vi "test_read-nmea-data2.vi"() -> ()   [LabVIEW 2019] (continued)
11,72,359,29,7*79\n\t\n15:13:14.60\tF9P\t$GAGSV,2,2,08,12,40,103,25,19,26,045,19,25,09,249,,36,26,308,17,7*71\n\t\n15:13:14.62\tF9P\t$GAGSV,2,1,08,02,08,297,,04,66,116,25,09,32,193,,11,72,359,,2*77\n\t\n15:13:14.64\tF9P\t$GAGSV,2,2,08,12,40,103,,19,26,045,,25,09,249,,36,26,308,,2*7D\n\t\n15:13:14.66\tF9P\t$GBGSV,1,1,04,11,49,132,31,14,87,114,29,28,,,21,33,61,220,31,1*44\n\t\n15:13:14.68\tF9P\t$GBGSV,1,1,03,11,49,132,28,14,87,114,,33,61,220,,3*49\n\t\n15:13:14.70\tF9P\t$GNGLL,3723.55651,N,12656.97723,E,061316.00,A,A*7D\n\t\n15:13:14.72\tF9P\t\t\n15:13:14.74\tF9P\t\t\n15:13:14.76\tF9P\t\t\n15:13:14.78\tF9P\t\t\n15:13:14.80\tF9P\t\t\n15:13:14.82\tF9P\t\t\n15:13:14.84\tF9P\t\t\n15:13:14.86\tF9P\t\t\n15:13:14.88\tF9P\t\t\n15:13:14.90\tF9P\t\t\n15:13:14.92\tF9P\t\t\n15:13:14.94\tF9P\t\t\n15:13:14.96\tF9P\t\t\n15:13:14.98\tF9P\t\t\n15:13:15.00\tF9P\t\t\n15:13:15.02\tF9P\t\t\n15:13:15.04\tF9P\t\t\n15:13:15.06\tF9P\t\t\n15:13:15.08\tF9P\t\t\n15:13:15.10\tF9P\t\t\n15:13:15.12\tF9P\t\t\n15:13:15.14\tF9P\t\t\n15:13:15.16\tF9P\t\t\n15:13:15.18\tF9P\t\t\n15:13:15.20\tF9P\t\t\n15:13:15.22\tF9P\t\t\n15:13:15.24\tF9P\t$GNRMC,061317.00,A,3723.55689,N,12656.97802,E,2.086,57.57,250720,,,A,V*36\n\t\n15:13:15.26\tF9P\t$GNVTG,57.57,T,,M,2.086,N,3.863,K,A*11\n\t\n15:13:15.28\tF9P\t$GNGGA,061317.00,3723.55689,N,12656.97802,E,1,12,0.86,49.2,M,18.5,M,,*7E\n\t\n15:13:15.30\tF9P\t$GNGSA,A,3,12,06,19,05,17,09,04,02,,,,,1.43,0.86,1.13,1*0B\n\t\n15:13:15.32\tF9P\t$GNGSA,A,3,85,70,71,84,,,,,,,,,1.43,0.86,1.13,2*09\n\t\n15:13:15.34\tF9P\t$GNGSA,A,3,36,19,11,04,09,12,,,,,,,1.43,0.86,1.13,3*0B\n\t\n15:13:15.36\tF9P\t$GNGSA,A,3,14,11,33,,,,,,,,,,1.43,0.86,1.13,4*0A\n\t\n15:13:15.38\tF9P\t$GPGSV,3,1,09,02,55,319,24,04,18,043,23,05,37,247,29,06,64,049,30,1*6A\n\t\n15:13:15.40\tF9P\t$GPGSV,3,2,09,09,45,074,36,12,23,276,22,17,33,154,36,19,52,157,32,1*6D\n\t\n15:13:15.42\tF9P\t$GPGSV,3,3,09,25,12,306,19,1*54\n\t\n15:13:15.44\tF9P\t$GPGSV,3,1,09,02,55,319,,04,18,043,16,05,37,247,24,06,64,049,23,6*62\n\t\n15:13:15.46\tF9P\t$GPGSV,3,2,09,09,45,074,27,12,23,276,,17,33,154,24,19,52,157,,6*68\n\t\n15:13:15.48\tF9P\t$GPGSV,3,3,09,25,12,306,,6*5B\n\t\n15:13:15.50\tF9P\t$GLGSV,2,1,08,69,11,031,25,70,70,038,24,71,53,206,39,72,05,210,21,1*7A\n\t\n15:13:15.52\tF9P\t$GLGSV,2,2,08,77,01,325,,84,19,123,17,85,70,070,32,86,37,330,,1*71\n\t\n15:13:15.54\tF9P\t$GLGSV,2,1,08,69,11,031,24,70,70,038,,71,53,206,26,72,05,210,,3*72\n\t\n15:13:15.56\tF9P\t$GLGSV,2,2,08,77,01,325,,84,19,123,19,85,70,070,20,86,37,330,,3*7E\n\t\n15:13:15.58\tF9P\t$GAGSV,2,1,08,02,08,297,08,04,66,116,24,09,32,193,33,11,72,359,29,7*70\n\t\n15:13:15.60\tF9P\t$GAGSV,2,2,08,12,40,103,26,19,26,045,18,25,09,249,,36,26,308,17,7*73\n\t\n15:13:15.62\tF9P\t$GAGSV,2,1,08,02,08,297,,04,66,116,,09,32,193,,11,72,359,,2*70\n\t\n15:13:15.64\tF9P\t$GAGSV,2,2,08,12,40,103,,19,26,045,,25,09,249,,36,26,308,,2*7D\n\t\n15:13:15.66\tF9P\t$GBGSV,1,1,04,11,49,132,30,14,87,114,28,28,,,21,33,61,220,32,1*47\n\t\n15:13:15.68\tF9P\t$GBGSV,1,1,03,11,49,132,26,14,87,114,,33,61,220,,3*47\n\t\n15:13:15.70\tF9P\t$GNGLL,3723.55689,N,12656.97802,E,061317.00,A,A*75\n\t\n15:13:15.72\tF9P\t\t\n15:13:15.74\tF9P\t\t\n15:13:15.76\tF9P\t\t\n15:13:15.78\tF9P\t\t\n15:13:15.80\tF9P\t\t\n15:13:15.82\tF9P\t\t\n15:13:15.84\tF9P\t\t\n15:13:15.86\tF9P\t\t\n15:13:15.88\tF9P\t\t\n15:13:15.90\tF9P\t\t\n15:13:15.92\tF9P\t\t\n15:13:15.94\tF9P\t\t\n15:13:15.96\tF9P\t\t\n15:13:15.98\tF9P\t\t\n15:13:16.00\tF9P\t\t\n15:13:16.02\tF9P\t\t\n15:13:16.04\tF9P\t\t\n15:13:16.06\tF9P\t\t\n15:13:16.08\tF9P\t\t\n15:13:16.10\tF9P\t\t\n15:13:16.12\tF9P\t\t\n15:13:16.14\tF9P\t\t\n15:13:16.16\tF9P\t\t\n15:13:16.18\tF9P\t\t\n15:13:16.20\tF9P\t\t\n15:13:16.22\tF9P\t\t\n15:13:16.24\tF9P\t$GNRMC,061318.00,A,3723.55723,N,12656.97894,E,2.495,64.44,250720,,,A,V*33\n\t\n15:13:16.26\tF9P\t$GNVTG,64.44,T,,M,2.495,N,4.621,K,A*1A\n\t\n15:13:16.28\tF9P\t$GNGGA,061318.00,3723.55723,N,12656.97894,E,1,12,0.86,49.1,M,18.5,M,,*7C\n\t\n15:13:16.30\tF9P\t$GNGSA,A,3,12,06,19,05,17,09,04,02,,,,,1.43,0.86,1.13,1*0B\n\t\n15:13:16.32\tF9P\t$GNGSA,A,3,85,70,71,84,,,,,,,,,1.43,0.86,1.13,2*09\n\t\n15:13:16.34\tF9P\t$GNGSA,A,3,36,19,11,04,09,12,,,,,,,1.43,0.86,1.13,3*0B\n\t\n15:13:16.36\tF9P\t$GNGSA,A,3,14,11,33,,,,,,,,,,1.43,0.86,1.13,4*0A\n\t\n15:13:16.38\tF9P\t$GPGSV,3,1,09,02,55,319,23,04,18,043,24,05,37,247,36,06,64,049,30,1*64\n\t\n15:13:16.40\tF9P\t$GPGSV,3,2,09,09,45,074,33,12,23,276,31,17,33,154,38,19,52,157,32,1*64\n\t\n15:13:16.42\tF9P\t$GPGSV,3,3,09,25,12,306,19,1*54\n\t\n15:13:16.44\tF9P\t$GPGSV,3,1,09,02,55,319,,04,18,043,15,05,37,247,24,06,64,049,23,6*61\n\t\n15:13:16.46\tF9P\t$GPGSV,3,2,09,09,45,074,28,12,23,276,26,17,33,154,30,19,52,157,,6*66\n\t\n15:13:16.48\tF9P\t$GPGSV,3,3,09,25,12,306,,6*5B\n\t\n15:13:16.50\tF9P\t$GLGSV,2,1,08,69,11,031,24,70,70,038,24,71,53,206,41,72,05,210,20,1*75\n\t\n15:13:16.52\tF9P\t$GLGSV,2,2,08,77,01,325,,84,19,123,11,85,70,070,31,86,37,330,,1*74\n\t\n15:13:16.54\tF9P\t$GLGSV,2,1,08,69,11,031,23,70,70,038,,71,53,206,26,72,05,210,,3*75\n\t\n15:13:16.56\tF9P\t$GLGSV,2,2,08,77,01,325,,84,19,123,18,85,70,070,23,86,37,330,,3*7C\n\t\n15:13:16.58\tF9P\t$GAGSV,2,1,08,02,08,297,11,04,66,116,30,09,32,193,39,11,72,359,32,7*7D\n\t\n15:13:16.60\tF9P\t$GAGSV,2,2,08,12,40,103,26,19,26,045,18,25,09,249,,36,26,308,18,7*7C\n\t\n15:13:16.62\tF9P\t$GAGSV,2,1,08,02,08,297,,04,66,116,,09,32,193,,11,72,359,,2*70\n\t\n15:13:16.64\tF9P\t$GAGSV,2,2,08,12,40,103,,19,26,045,,25,09,249,,36,26,308,,2*7D\n\t\n15:13:16.66\tF9P\t$GBGSV,1,1,04,11,49,132,30,14,87,114,27,28,,,22,33,61,220,27,1*4F\n\t\n15:13:16.68\tF9P\t$GBGSV,1,1,03,11,49,132,,14,87,114,,33,61,220,,3*43\n\t\n15:13:16.70\tF9P\t$GNGLL,3723.55723,N,12656.97894,E,061318.00,A,A*74\n\t\n15:13:16.72\tF9P\t\t\n15:13:16.74\tF9P\t\t\n15:13:16.76\tF9P\t\t\n15:13:16.78\tF9P\t\t\n15:13:16.80\tF9P\t\t\n15:13:16.82\tF9P\t\t\n15:13:16.84\tF9P\t\t\n15:13:16.86\tF9P\t\t\n15:13:16.88\tF9P\t\t\n15:13:16.90\tF9P\t\t\n15:13:16.92\tF9P\t\t\n15:13:16.94\tF9P\t\t\n15:13:16.96\tF9P\t\t\n15:13:16.98\tF9P\t\t\n15:13:17.00\tF9P\t\t\n15:13:17.02\tF9P\t\t\n15:13:17.04\tF9P\t\t\n15:13:17.06\tF9P\t\t\n15:13:17.08\tF9P\t\t\n15:13:17.10\tF9P\t\t\n15:13:17.12\tF9P\t\t\n15:13:17.14\tF9P\t\t\n15:13:17.16\tF9P\t\t\n15:13:17.18\tF9P\t\t\n15:13:17.20\tF9P\t\t\n15:13:17.22\tF9P\t\t\n15:13:17.24\tF9P\t$GNRMC,061319.00,A,3723.55735,N,12656.97964,E,1.814,63.78,250720,,,A,V*35\n\t\n15:13:17.26\tF9P\t$GNVTG,63.78,T,,M,1.814,N,3.359,K,A*19\n\t\n15:13:17.28\tF9P\t$GNGGA,061319.00,3723.55735,N,12656.97964,E,1,12,0.88,50.1,M,18.5,M,,*72\n\t\n15:13:17.30\tF9P\t$GNGSA,A,3,12,06,19,05,17,09,04,02,,,,,1.43,0.88,1.14,1*02\n\t\n15:13:17.32\tF9P\t$GNGSA,A,3,85,70,71,84,,,,,,,,,1.43,0.88,1.14,2*00\n\t\n15:13:17.34\tF9P\t$GNGSA,A,3,36,19,11,04,09,12,,,,,,,1.43,0.88,1.14,3*02\n\t\n15:13:17.36\tF9P\t$GNGSA,A,3,14,11,33,,,,,,,,,,1.43,0.88,1.14,4*03\n\t\n15:13:17.38\tF9P\t$GPGSV,3,1,09,02,55,319,23,04,18,043,26,05,37,247,33,06,64,049,24,1*66\n\t\n15:13:17.40\tF9P\t$GPGSV,3,2,09,09,45,074,34,12,23,276,25,17,33,154,35,19,52,157,31,1*68\n\t\n15:13:17.42\tF9P\t$GPGSV,3,3,09,25,12,306,18,1*55\n\t\n15:13:17.44\tF9P\t$GPGSV,3,1,09,02,55,319,,04,18,043,14,05,37,247,24,06,64,049,23,6*60\n\t\n15:13:17.46\tF9P\t$GPGSV,3,2,09,09,45,074,28,12,23,276,27,17,33,154,25,19,52,157,,6*63\n\t\n15:13:17.48\tF9P\t$GPGSV,3,3,09,25,12,306,,6*5B\n\t\n15:13:17.50\tF9P\t$GLGSV,2,1,08,69,11,031,24,70,70,038,24,71,53,206,36,72,05,210,20,1*75\n\t\n15:13:17.52\tF9P\t$GLGSV,2,2,08,77,01,325,,84,19,123,12,85,70,070,31,86,37,330,,1*77\n\t\n15:13:17.54\tF9P\t$GLGSV,2,1,08,69,11,031,24,70,70,038,,71,53,206,36,72,05,210,,3*73\n\t\n15:13:17.56\tF9P\t$GLGSV,2,2,08,77,01,325,,84,19,123,19,85,70,070,23,86,37,330,,3*7D\n\t\n15:13:17.58\tF9P\t$GAGSV,2,1,08,02,08,297,08,04,66,116,31,09,32,193,38,11,72,359,35,7*72\n\t\n15:13:17.60\tF9P\t$GAGSV,2,2,08,12,40,103,31,19,26,045,17,25,09,249,,36,26,308,20,7*7E\n\t\n15:13:17.62\tF9P\t$GAGSV,2,1,08,02,08,297,,04,66,116,,09,32,193,,11,72,359,,2*70\n\t\n15:13:17.64\tF9P\t$GAGSV,2,2,08,12,40,103,,19,26,045,,25,09,249,,36,26,308,,2*7D\n\t\n15:13:17.66\tF9P\t$GBGSV,1,1,04,11,49,132,29,14,87,114,32,28,,,22,33,61,220,29,1*4D\n\t\n15:13:17.68\tF9P\t$GBGSV,1,1,03,11,49,132,29,14,87,114,,33,61,220,,3*48\n\t\n15:13:17.70\tF9P\t$GNGLL,3723.55735,N,12656.97964,E,061319.00,A,A*7C\n\t\n15:13:17.72\tF9P\t\t\n15:13:17.74\tF9P\t\t\n15:13:17.76\tF9P\t\t\n15:13:17.78\tF9P\t\t\n15:13:17.80\tF9P\t\t\n15:13:17.82\tF9P\t\t\n15:13:17.84\tF9P\t\t\n15:13:17.86\tF9P\t\t\n15:13:17.88\tF9P\t\t\n15:13:17.90\tF9P\t\t\n15:13:17.92\tF9P\t\t\n15:13:17.94\tF9P\t\t\n15:13:17.96\tF9P\t\t\n15:13:17.98\tF9P\t\t\n15:13:18.00\tF9P\t\t\n15:13:18.02\tF9P\t\t\n15:13:18.04\tF9P\t\t\n15:13:18.06\tF9P\t\t\n15:13:18.08\tF9P\t\t\n15:13:18.10\tF9P\t\t\n15:13:18.12\tF9P\t\t\n15:13:18.14\tF9P\t\t\n15:13:18.16\tF9P\t\t\n15:13:18.18\tF9P\t\t\n15:13:18.20\tF9P\t\t\n15:13:18.22\tF9P\t\t\n15:13:18.24\tF9P\t$GNRMC,061320.00,A,3723.55750,N,12656.98041,E,1.847,68.01,250720,,,A,V*3E\n\t\n15:13:18.26\tF9P\t$GNVTG,68.01,T,,M,1.847,N,3.421,K,A*12\n\t\n15:13:18.28\tF9P\t$GNGGA,061320.00,3723.55750,N,12656.98041,E,1,12,0.72,49.8,M,18.5,M,,*7E\n\t\n15:13:18.30\tF9P\t$GNGSA,A,3,12,06,19,05,17,09,04,02,,,,,1.23,0.72,0.99,1*05\n\t\n15:13:18.32\tF9P\t$GNGSA,A,3,85,70,71,84,,,,,,,,,1.23,0.72,0.99,2*07\n\t\n15:13:18.34\tF9P\t$GNGSA,A,3,36,19,11,04,09,12,,,,,,,1.23,0.72,0.99,3*05\n\t\n15:13:18.36\tF9P\t$GNGSA,A,3,14,11,33,,,,,,,,,,1.23,0.72,0.99,4*04\n\t\n15:13:18.38\tF9P\t$GPGSV,3,1,09,02,55,320,23,04,18,043,24,05,37,247,35,06,64,049,25,1*69\n\t\n15:13:18.40\tF9P\t$GPGSV,3,2,09,09,45,074,37,12,23,276,32,17,33,154,36,19,52,157,30,1*6F\n\t\n15:13:18.42\tF9P\t$GPGSV,3,3,09,25,12,306,18,1*55\n\t\n15:13:18.44\tF9P\t$GPGSV,3,1,09,02,55,320,,04,18,043,14,05,37,247,21,06,64,049,25,6*69\n\t\n15:13:18.46\tF9P\t$GPGSV,3,2,09,09,45,074,28,12,23,276,27,17,33,154,22,19,52,157,,6*64\n\t\n15:13:18.48\tF9P\t$GPGSV,3,3,09,25,12,306,,6*5B\n\t\n15:13:18.50\tF9P\t$GLGSV,2,1,08,69,11,031,31,70,70,038,25,71,53,206,45,72,05,210,19,1*7E\n\t\n15:13:18.52\tF9P\t$GLGSV,2,2,08,77,01,325,,84,19,123,10,85,70,070,25,86,37,330,,1*70\n\t\n15:13:18.54\tF9P\t$GLGSV,2,1,08,69,11,031,23,70,70,038,,71,53,206,28,72,05,210,,3*7B\n\t\n15:13:18.56\tF9P\t$GLGSV,2,2,08,77,01,325,,84,19,123,19,85,70,070,23,86,37,330,,3*7D\n\t\n15:13:18.58\tF9P\t$GAGSV,2,1,08,02,08,297,12,04,66,116,26,09,32,193,36,11,72,359,27,7*72\n\t\n15:13:18.60\tF9P\t$GAGSV,2,2,08,12,40,103,26,19,26,045,17,25,09,249,,36,26,308,19,7*72\n\t\n15:13:18.62\tF9P\t$GAGSV,2,1,08,02,08,297,,04,66,116,,09,32,193,33,11,72,359,,2*70\n\t\n15:13:18.64\tF9P\t$GAGSV,2,2,08,12,40,103,,19,26,045,,25,09,249,,36,26,308,,2*7D\n\t\n15:13:18.66\tF9P\t$GBGSV,1,1,04,11,49,132,29,14,87,114,31,28,,,23,33,61,220,33,1*44\n\t\n15:13:18.68\tF9P\t$GBGSV,1,1,03,11,49,132,24,14,87,114,,33,61,220,,3*45\n\t\n15:13:18.70\tF9P\t$GNGLL,3723.55750,N,12656.98041,E,061320.00,A,A*74\n\t\n15:13:18.72\tF9P\t\t\n15:13:18.74\tF9P\t\t\n15:13:18.76\tF9P\t\t\n15:13:18.78\tF9P\t\t\n15:13:18.80\tF9P\t\t\n15:13:18.82\tF9P\t\t\n15:13:18.84\tF9P\t\t\n15:13:18.86\tF9P\t\t\n15:13:18.88\tF9P\t\t\n15:13:18.90\tF9P\t\t\n15:13:18.92\tF9P\t\t\n15:13:18.94\tF9P\t\t\n15:13:18.96\tF9P\t\t\n15:13:18.98\tF9P\t\t\n15:13:19.00\tF9P\t\t\n15:13:19.02\tF9P\t\t\n15:13:19.04\tF9P\t\t\n15:13:19.06\tF9P\t\t\n15:13:19.08\tF9P\t\t\n15:13:19.10\tF9P\t\t\n15:13:19.12\tF9P\t\t\n15:13:19.14\tF9P\t\t\n15:13:19.16\tF9P\t\t\n15:13:19.18\tF9P\t\t\n15:13:19.20\tF9P\t\t\n15:13:19.22\tF9P\t\t\n15:13:19.24\tF9P\t$GNRMC,061321.00,A,3723.55771,N,12656.98117,E,1.921,64.56,250720,,,A,V*31\n\t\n15:13:19.26\tF9P\t$GNVTG,64.56,T,,M,1.921,N,3.558,K,A*12\n\t\n15:13:19.28\tF9P\t$GNGGA,061321.00,3723.55771,N,12656.98117,E,1,12,0.72,49.7,M,18.5,M,,*71\n\t\n15:13:19.30\tF9P\t$GNGSA,A,3,12,06,19,05,17,09,04,02,,,,,1.23,0.72,0.99,1*05\n\t\n15:13:19.32\tF9P\t$GNGSA,A,3,85,70,71,84,,,,,,,,,1.23,0.72,0.99,2*07\n\t\n15:13:19.34\tF9P\t$GNGSA,A,3,36,19,11,04,09,12,,,,,,,1.23,0.72,0.99,3*05\n\t\n15:13:19.36\tF9P\t$GNGSA,A,3,14,11,33,,,,,,,,,,1.23,0.72,0.99,4*04\n\t\n15:13:19.38\tF9P\t$GPGSV,3,1,09,02,55,320,24,04,18,043,25,05,37,247,29,06,64,049,28,1*6F\n\t\n15:13:19.40\tF9P\t$GPGSV,3,2,09,09,45,074,30,12,23,276,35,17,33,154,37,19,52,157,32,1*6C\n\t\n15:13:19.42\tF9P\t$GPGSV,3,3,09,25,12,306,19,1*54\n\t\n15:13:19.44\tF9P\t$GPGSV,3,1,09,02,55,320,,04,18,043,16,05,37,247,21,06,64,049,27,6*69\n\t\n15:13:19.46\tF9P\t$GPGSV,3,2,09,09,45,074,28,12,23,276,28,17,33,154,29,19,52,157,,6*60\n\t\n15:13:19.48\tF9P\t$GPGSV,3,3,09,25,12,306,,6*5B\n\t\n15:13:19.50\tF9P\t$GLGSV,2,1,08,69,11,031,32,70,70,038,25,71,53,206,41,72,05,210,20,1*73\n\t\n15:13:19.52\tF9P\t$GLGSV,2,2,08,77,01,325,,84,19,123,11,85,70,070,34,86,37,330,,1*71\n\t\n15:13:19.54\tF9P\t$GLGSV,2,1,08,69,11,031,23,70,70,038,,71,53,206,27,72,05,210,,3*74\n\t\n15:13:19.56\tF9P\t$GLGSV,2,2,08,77,01,325,,84,19,123,19,85,70,070,24,86,37,330,,3*7A\n\t\n15:13:19.58\tF9P\t$GAGSV,2,1,08,02,08,297,08,04,66,116,25,09,32,193,40,11,72,359,25,7*79\n\t\n15:13:19.60\tF9P\t$GAGSV,2,2,08,12,40,103,26,19,26,045,17,25,09,249,,36,26,308,20,7*78\n\t\n15:13:19.62\tF9P\t$GAGSV,2,1,08,02,08,297,,04,66,116,,09,32,193,34,11,72,359,,2*77\n\t\n15:13:19.64\tF9P\t$GAGSV,2,2,08,12,40,103,,19,26,045,,25,09,249,,36,26,308,,2*7D\n\t\n15:13:19.66\tF9P\t$GBGSV,1,1,04,11,49,132,31,14,87,114,31,28,,,23,33,61,220,36,1*48\n\t\n15:13:19.68\tF9P\t$GBGSV,1,1,03,11,49,132,34,14,87,114,,33,61,220,,3*44\n\t\n15:13:19.70\tF9P\t$GNGLL,3723.55771,N,12656.98117,E,061321.00,A,A*74\n\t\n15:13:19.72\tF9P\t\t\n15:13:19.74\tF9P\t\t\n15:13:19.76\tF9P\t\t\n15:13:19.78\tF9P\t\t\n15:13:19.80\tF9P\t\t\n15:13:19.82\tF9P\t\t\n15:13:19.84\tF9P\t\t\n15:13:19.86\tF9P\t\t\n15:13:19.88\tF9P\t\t\n15:13:19.90\tF9P\t\t\n15:13:19.92\tF9P\t\t\n15:13:19.94\tF9P\t\t\n15:13:19.96\tF9P\t\t\n15:13:19.98\tF9P\t\t\n15:13:20.00\tF9P\t\t\n15:13:20.02\tF9P\t\t\n15:13:20.04\tF9P\t\t\n15:13:20.06\tF9P\t\t\n15:13:20.08\tF9P\t\t\n15:13:20.10\tF9P\t\t\n15:13:20.12\tF9P\t\t\n15:13:20.14\tF9P\t\t\n15:13:20.16\tF9P\t\t\n15:13:20.18\tF9P\t\t\n15:13:20.20\tF9P\t\t\n15:13:20.22\tF9P\t\t\n15:13:20.24\tF9P\t$GNRMC,061322.00,A,3723.55823,N,12656.98186,E,2.122,59.10,250720,,,A,V*36\n\t\n15:13:20.26\tF9P\t$GNVTG,59.10,T,,M,2.122,N,3.930,K,A*14\n\t\n15:13:20.28\tF9P\t$GNGGA,061322.00,3723.55823,N,12656.98186,E,1,12,0.86,49.2,M,18.5,M,,*7C\n\t\n15:13:20.30\tF9P\t$GNGSA,A,3,12,06,19,05,17,09,04,02,,,,,1.42,0.86,1.13,1*0A\n\t\n15:13:20.32\tF9P\t$GNGSA,A,3,85,70,71,84,,,,,,,,,1.42,0.86,1.13,2*08\n\t\n15:13:20.34\tF9P\t$GNGSA,A,3,36,19,11,04,09,12,,,,,,,1.42,0.86,1.13,3*0A\n\t\n15:13:20.36\tF9P\t$GNGSA,A,3,14,11,33,,,,,,,,,,1.42,0.86,1.13,4*0B\n\t\n15:13:20.38\tF9P\t$GPGSV,3,1,09,02,55,320,25,04,17,043,25,05,37,247,31,06,64,049,33,1*62\n\t\n15:13:20.40\tF9P\t$GPGSV,3,2,09,09,45,074,35,12,23,276,31,17,33,154,35,19,52,157,33,1*6E\n\t\n15:13:20.42\tF9P\t$GPGSV,3,3,09,25,12,306,20,1*5E\n\t\n15:13:20.44\tF9P\t$GPGSV,3,1,09,02,55,320,,04,17,043,15,05,37,247,23,06,64,049,33,6*62\n\t\n15:13:20.46\tF9P\t$GPGSV,3,2,09,09,45,074,33,12,23,276,27,17,33,154,29,19,52,157,,6*65\n\t\n15:13:20.48\tF9P\t$GPGSV,3,3,09,25,12,306,,6*5B\n\t\n15:13:20.50\tF9P\t$GLGSV,2,1,08,69,11,031,33,70,70,038,25,71,53,206,39,72,05,210,20,1*7D\n\t\n15:13:20.52\tF9P\t$GLGSV,2,2,08,77,01,325,,84,19,123,12,85,70,070,26,86,37,330,,1*71\n\t\n15:13:20.54\tF9P\t$GLGSV,2,1,08,69,11,031,24,70,70,038,,71,53,206,28,72,05,210,,3*7C\n\t\n15:13:20.56\tF9P\t$GLGSV,2,2,08,77,01,325,,84,19,123,19,85,70,070,23,86,37,330,,3*7D\n\t\n15:13:20.58\tF9P\t$GAGSV,2,1,08,02,08,297,08,04,66,116,26,09,32,193,38,11,72,359,26,7*76\n\t\n15:13:20.60\tF9P\t$GAGSV,2,2,08,12,40,103,31,19,26,045,18,25,09,249,,36,26,308,20,7*71\n\t\n15:13:20.62\tF9P\t$GAGSV,2,1,08,02,08,297,,04,66,116,,09,32,193,31,11,72,359,,2*72\n\t\n15:13:20.64\tF9P\t$GAGSV,2,2,08,12,40,103,,19,26,045,,25,09,249,,36,26,308,,2*7D\n\t\n15:13:20.66\tF9P\t$GBGSV,1,1,04,11,49,132,30,14,87,114,29,28,,,22,33,61,220,33,1*44\n\t\n15:13:20.68\tF9P\t$GBGSV,1,1,03,11,49,132,30,14,87,114,,33,61,220,,3*40\n\t\n15:13:20.70\tF9P\t$GNGLL,3723.55823,N,12656.98186,E,061322.00,A,A*77\n\t\n15:13:20.72\tF9P\t\t\n15:13:20.74\tF9P\t\t\n15:13:20.76\tF9P\t\t\n15:13:20.78\tF9P\t\t\n15:13:20.80\tF9P\t\t\n15:13:20.82\tF9P\t\t\n15:13:20.84\tF9P\t\t\n15:13:20.86\tF9P\t\t\n15:13:20.88\tF9P\t\t\n15:13:20.90\tF9P\t\t\n15:13:20.92\tF9P\t\t\n15:13:20.94\tF9P\t\t\n15:13:20.96\tF9P\t\t\n15:13:20.98\tF9P\t\t\n15:13:21.00\tF9P\t\t\n15:13:21.02\tF9P\t\t\n15:13:21.04\tF9P\t\t\n15:13:21.06\tF9P\t\t\n15:13:21.08\tF9P\t\t\n15:13:21.10\tF9P\t\t\n15:13:21.12\tF9P\t\t\n15:13:21.14\tF9P\t\t\n15:13:21.16\tF9P\t\t\n15:13:21.18\tF9P\t\t\n15:13:21.20\tF9P\t\t\n15:13:21.22\tF9P\t\t\n15:13:21.24\tF9P\t$GNRMC,061323.00,A,3723.55859,N,12656.98249,E,1.864,50.09,250720,,,A,V*33\n\t\n15:13:21.26\tF9P\t$GNVTG,50.09,T,,M,1.864,N,3.451,K,A*17\n\t\n15:13:21.28\tF9P\t$GNGGA,061323.00,3723.55859,N,12656.98249,E,1,12,0.73,49.6,M,18.5,M,,*7E\n\t\n15:13:21.30\tF9P\t$GNGSA,A,3,12,06,19,05,17,09,04,02,,,,,1.24,0.73,1.00,1*02\n\t\n15:13:21.32\tF9P\t$GNGSA,A,3,85,70,71,84,,,,,,,,,1.24,0.73,1.00,2*00\n\t\n15:13:21.34\tF9P\t$GNGSA,A,3,36,19,11,04,09,12,,,,,,,1.24,0.73,1.00,3*02\n\t\n15:13:21.36\tF9P\t$GNGSA,A,3,14,11,33,,,,,,,,,,1.24,0.73,1.00,4*03\n\t\n15:13:21.38\tF9P\t$GPGSV,3,1,09,02,55,320,25,04,17,043,24,05,38,248,35,06,64,049,32,1*66\n\t\n15:13:21.40\tF9P\t$GPGSV,3,2,09,09,45,074,29,12,23,276,35,17,33,154,32,19,52,157,30,1*63\n\t\n15:13:21.42\tF9P\t$GPGSV,3,3,09,25,12,306,21,1*5F\n\t\n15:13:21.44\tF9P\t$GPGSV,3,1,09,02,55,320,,04,17,043,18,05,38,248,22,06,64,049,33,6*6E\n\t\n15:13:21.46\tF9P\t$GPGSV,3,2,09,09,45,074,30,12,23,276,27,17,33,154,28,19,52,157,,6*67\n\t\n15:13:21.48\tF9P\t$GPGSV,3,3,09,25,12,306,,6*5B\n\t\n15:13:21.50\tF9P\t$GLGSV,2,1,08,69,11,031,29,70,70,038,25,71,53,206,37,72,05,210,20,1*78\n\t\n15:13:21.52\tF9P\t$GLGSV,2,2,08,77,01,325,,84,19,123,12,85,70,070,32,86,37,330,,1*74\n\t\n15:13:21.54\tF9P\t$GLGSV,2,1,08,69,11,031,25,70,70,038,,71,53,206,27,72,05,210,,3*72\n\t\n15:13:21.56\tF9P\t$GLGSV,2,2,08,77,01,325,,84,19,123,18,85,70,070,24,86,37,330,,3*7B\n\t\n15:13:21.58\tF9P\t$GAGSV,2,1,08,02,08,297,10,04,66,116,30,09,32,193,38,11,72,359,26,7*78\n\t\n15:13:21.60\tF9P\t$GAGSV,2,2,08,12,40,103,32,19,26,045,18,25,09,249,,36,26,308,21,7*73\n\t\n15:13:21.62\tF9P\t$GAGSV,2,1,08,02,08,297,,04,66,116,,09,32,193,34,11,72,359,,2*77\n\t\n15:13:21.64\tF9P\t$GAGSV,2,2,08,12,40,103,,19,26,045,,25,09,249,,36,26,308,,2*7D\n\t\n15:13:21.66\tF9P\t$GBGSV,1,1,04,11,49,132,34,14,87,114,29,28,,,29,33,61,220,36,1*4E\n\t\n15:13:21.68\tF9P\t$GBGSV,1,1,03,11,49,132,,14,87,114,,33,61,220,,3*43\n\t\n15:13:21.70\tF9P\t$GNGLL,3723.55859,N,12656.98249,E,061323.00,A,A*7B\n\t\n15:13:21.72\tF9P\t\t\n15:13:21.74\tF9P\t\t\n15:13:21.76\tF9P\t\t\n15:13:21.78\tF9P\t\t\n15:13:21.80\tF9P\t\t\n15:13:21.82\tF9P\t\t\n15:13:21.84\tF9P\t\t\n15:13:21.86\tF9P\t\t\n15:13:21.88\tF9P\t\t\n15:13:21.90\tF9P\t\t\n15:13:21.92\tF9P\t\t\n15:13:21.94\tF9P\t\t\n15:13:21.96\tF9P\t\t\n15:13:21.98\tF9P\t\t\n15:13:22.00\tF9P\t\t\n15:13:22.02\tF9P\t\t\n15:13:22.04\tF9P\t\t\n15:13:22.06\tF9P\t\t\n15:13:22.08\tF9P\t\t\n15:13:22.10\tF9P\t\t\n15:13:22.12\tF9P\t\t\n15:13:22.14\tF9P\t\t\n15:13:22.16\tF9P\t\t\n15:13:22.18\tF9P\t\t\n15:13:22.20\tF9P\t\t\n15:13:22.22\tF9P\t\t\n15:13:22.24\tF9P\t$GNRMC,061324.00,A,3723.55902,N,12656.98306,E,1.996,45.57,250720,,,A,V*32\n\t\n15:13:22.26\tF9P\t$GNVTG,45.57,T,,M,1.996,N,3.696,K,A*1D\n\t\n15:13:22.28\tF9P\t$GNGGA,061324.00,3723.55902,N,12656.98306,E,1,12,0.89,50.0,M,18.5,M,,*77\n\t\n15:13:22.30\tF9P\t$GNGSA,A,3,12,06,19,05,17,09,04,02,,,,,1.44,0.89,1.13,1*03\n\t\n15:13:22.32\tF9P\t$GNGSA,A,3,85,70,71,84,,,,,,,,,1.44,0.89,1.13,2*01\n\t\n15:13:22.34\tF9P\t$GNGSA,A,3,36,19,11,04,09,12,,,,,,,1.44,0.89,1.13,3*03\n\t\n15:13:22.36\tF9P\t$GNGSA,A,3,14,11,33,,,,,,,,,,1.44,0.89,1.13,4*02\n\t\n15:13:22.38\tF9P\t$GPGSV,3,1,09,02,55,320,32,04,17,043,23,05,38,248,35,06,64,050,33,1*6E\n\t\n15:13:22.40\tF9P\t$GPGSV,3,2,09,09,45,074,28,12,23,276,39,17,33,154,32,19,52,157,33,1*6D\n\t\n15:13:22.42\tF9P\t$GPGSV,3,3,09,25,12,306,22,1*5C\n\t\n15:13:22.44\tF9P\t$GPGSV,3,1,09,02,55,320,,04,17,043,17,05,38,248,
